vi "Save Process Data TypeDef.vi"(8 "error in (no error)":errorcluster, 10 "Path to Library":path, 11 "ProcessData Ref":refnum<vi>) -> (0 "error out":errorcluster)   [LabVIEW 2020]
panel:
  out "Error Out":errorcluster
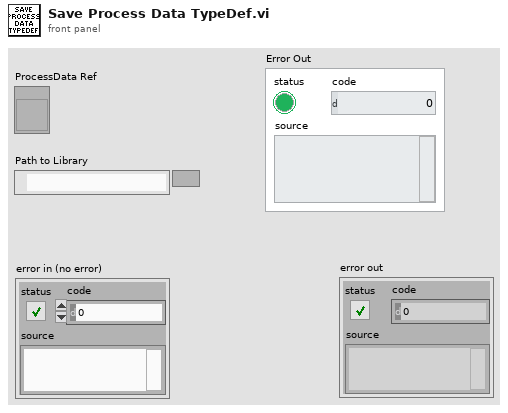
[diagram p1: front panel]
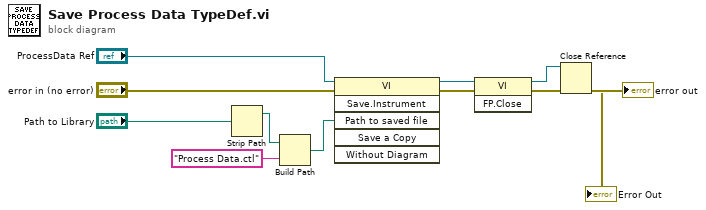
[diagram p0: block diagram]
diagram:
  n1 = Strip Path(path="Path to Library") -> (stripped path=w11:path)  [unwired: 1 out]
  n2 = Build Path(base path=w11, name or relative path="Process Data.ctl") -> (appended path=w6:path)
  n3 = invoke class="VI" method="Save.Instrument"(reference="ProcessData Ref", error in="error in (no error)", "Path to saved file"=w6) -> (reference out=w5:refnum<vi>, error out=→"Error Out":errorcluster)  [unwired: 3 in, 4 out]
  n4 = invoke class="VI" method="FP.Close"(reference=w5) -> (reference out=w3:refnum<vi>, error out=w4:errorcluster)  [unwired: 2 in, 1 out]
  n5 = Close Reference(reference=w3, error in (no error)=w4) -> (error out=→"error out":errorcluster)
